vi "Exit Structure.vi"(0 "Diagram in":refnum<vi>, 5 "Outputs":refnum<vi>[](array[refnum]), 11 "error in (no error)":errorcluster) -> (4 "Diagram out":refnum<vi>, 6 "Outputs":refnum<vi>[](array[refnum]), 15 "error out":errorcluster)   [LabVIEW 2015, in "Scripting.lvlib"]
uses:
  Scripting.lvlib
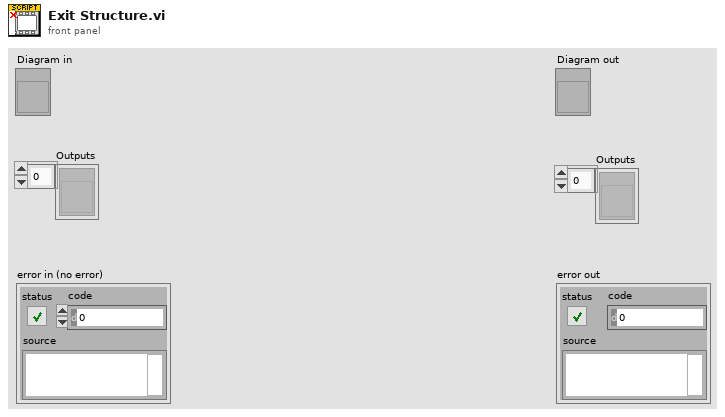
[diagram p1: front panel]
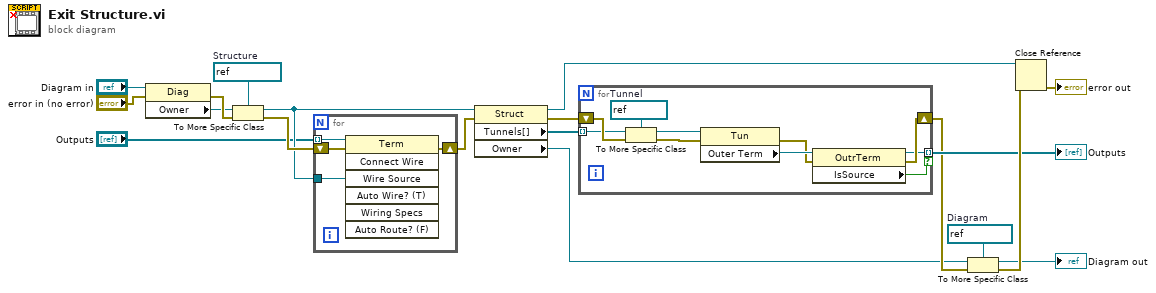
[diagram p0: block diagram]
diagram:
  w14 = refnum<vi> refnum  # Diagram
  w17 = refnum<vi> refnum  # Structure
  n1 = property class="Diag"(reference="Diagram in", error in="error in (no error)") -> (error out=w18:errorcluster, "Owner"=w16:refnum<vi>)  [unwired: 1 out]
  n2 = To More Specific Class(target class=w17, reference=w16, error in=w18) -> (specific class reference=w13:refnum<vi>, error out=w19:errorcluster)
  n3 = for {
    tunnel: w13 -> [w22]
    shift-right: [w21] -> w12
    shift-left: w19 -> [w23]
    tunnel: "Outputs" -> [w20] mode=indexing
    n4 = invoke class="Term" method="Connect Wire"(reference=w20, error in=w23, "Wire Source"=w22) -> (error out=w21:errorcluster)  [unwired: 4 in, 6 out]
  }
  n5 = property class="Struct"(reference=w13, error in=w12) -> (reference out=w1:refnum<vi>, error out=w2:errorcluster, "Tunnels[]"=w3:refnum<vi>[], "Owner"=w4:refnum<vi>)
  n6 = for {
    tunnel: w3 -> [w26] mode=indexing
    tunnel: [w28] -> w7 mode=indexing if=w29
    shift-right: [w30] -> w6
    shift-left: w2 -> [w33]
    w24 = refnum<vi> refnum  # Tunnel
    n7 = To More Specific Class(target class=w24, reference=w26, error in=w33) -> (specific class reference=w25:refnum<vi>, error out=w27:errorcluster)
    n8 = property class="Tun"(reference=w25, error in=w27) -> (error out=w31:errorcluster, "Outer Term"=w32:refnum<vi>)  [unwired: 1 out]
    n9 = property class="OutrTerm"(reference=w32, error in=w31) -> (reference out=w28:refnum<vi>, error out=w30:errorcluster, "IsSource"=w29:bool)
  }
  "Outputs" <- w7
  n10 = To More Specific Class(target class=w14, reference=w4, error in=w6) -> (specific class reference=→"Diagram out":refnum<vi>, error out=w15:errorcluster)
  n11 = Close Reference(reference=w1, error in (no error)=w15) -> (error out=→"error out":errorcluster)
